vi "Testing.vi"() -> ()   [LabVIEW 2011]
uses:
  Sliding Menu Library/Sliding Menu xControl/Sliding Menu XControl.xctl
  <vilib>/Utility/cursorutil.llb/Set Cursor (Icon Pict).vi
panel:
  in  "Space Between Buttons":i32=3
  in  "Number of Buttons":i32=6
  in  "Sliding Menu XControl":i32(xcontrol)
  in  "Up":bool
  in  "Down":bool
  in  "stop":bool
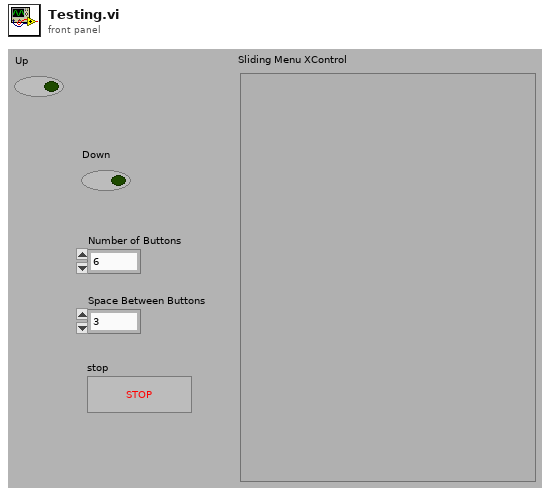
[diagram p1: front panel]
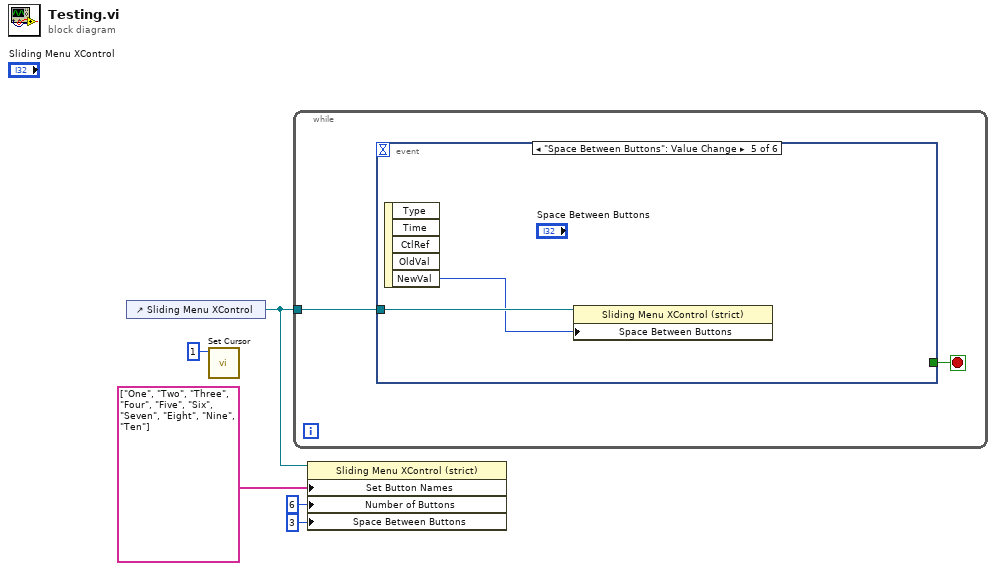
[diagram p0: block diagram]
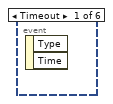
[diagram p2: hidden frame]
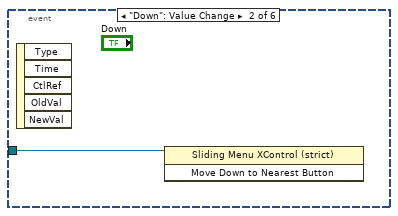
[diagram p3: hidden frame]
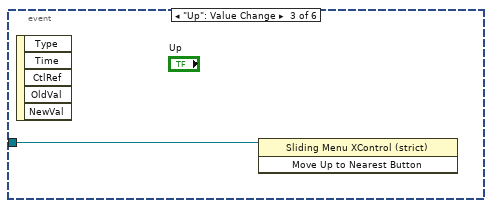
[diagram p4: hidden frame]
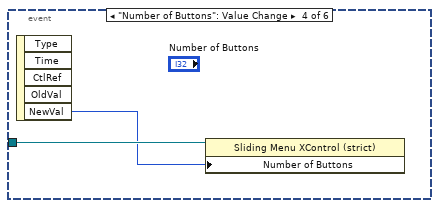
[diagram p5: hidden frame]
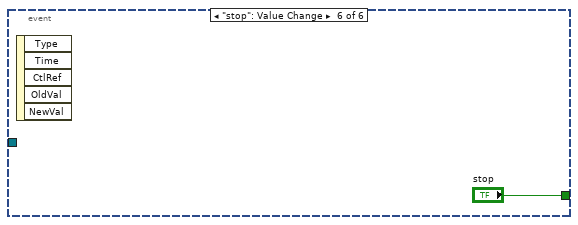
[diagram p6: hidden frame]
diagram:
  n1 = control-ref of="Sliding Menu XControl"() -> (w4:refnum<vi>)
  n2 = call-poly <vilib>:"Set Cursor.vi"("icon"=u16 1) -> ()  [unwired: 9 in, 2 out]
  n3 = while {
    tunnel: w4 -> [w6]
    stop <- w7 stop-if-true
    n4 = event shown="[4] \"Space Between Buttons\": Value Change" {
      selector: _ -> [_ _ _ _ _ _]
      dyn-events: _ -> [_ _ _ _ _ _]
      timeout: _ -> [_ _ _ _ _ _]
      tunnel: [_ _ _ _ _ "stop"] -> w7
      tunnel: w6 -> [_ w8 w9 w11 w13 _]
      event Timeout {
        n5 = event-data() -> ()  [unwired: 1 in, 2 out]
      }
      event "Down": Value Change {
        n6 = event-data() -> ()  [unwired: 1 in, 5 out]
        n7 = invoke class="Sliding Menu XControl (strict)" method="Move Down to Nearest Button"(reference=w8) -> ()  [unwired: 2 in, 3 out]
      }
      event "Up": Value Change {
        n8 = event-data() -> ()  [unwired: 1 in, 5 out]
        n9 = invoke class="Sliding Menu XControl (strict)" method="Move Up to Nearest Button"(reference=w9) -> ()  [unwired: 2 in, 3 out]
      }
      event "Number of Buttons": Value Change {
        n10 = event-data() -> ("NewVal"=w10:i32)  [unwired: 1 in, 4 out]
        n11 = property class="Sliding Menu XControl (strict)"(reference=w11, "Number of Buttons"=w10) -> ()  [unwired: 1 in, 2 out]
      }
      event "Space Between Buttons": Value Change {
        n12 = event-data() -> ("NewVal"=w12:i32)  [unwired: 1 in, 4 out]
        n13 = property class="Sliding Menu XControl (strict)"(reference=w13, "Space Between Buttons"=w12) -> ()  [unwired: 1 in, 2 out]
      }
      event "stop": Value Change {
        n14 = event-data() -> ()  [unwired: 1 in, 5 out]
      }
    }
  }
  n15 = property on="Property Node" class="Sliding Menu XControl (strict)"(reference=w4, "Set Button Names"=string[] ["One", "Two", "Three", "Four", "Five", "Six", "Seven", "Eight", "Nine", "Ten"], "Number of Buttons"=6, "Space Between Buttons"=3) -> ()  [unwired: 1 in, 2 out]
